vi "Clear Plugin.vi"(8 "error in (no error)":errorcluster, 10 "Plugin":string, 11 "Execution UI in":refnum<class "Execution UI.lvclass">) -> (0 "error out":errorcluster, 3 "Execution UI out":refnum<class "Execution UI.lvclass">)   [LabVIEW 2020, in "Execution UI.lvclass"]
uses:
  Execution UI.lvclass
  Execution UI.lvclass/Execution UI.ctl
  Framework/Plugin/Plugin.lvclass
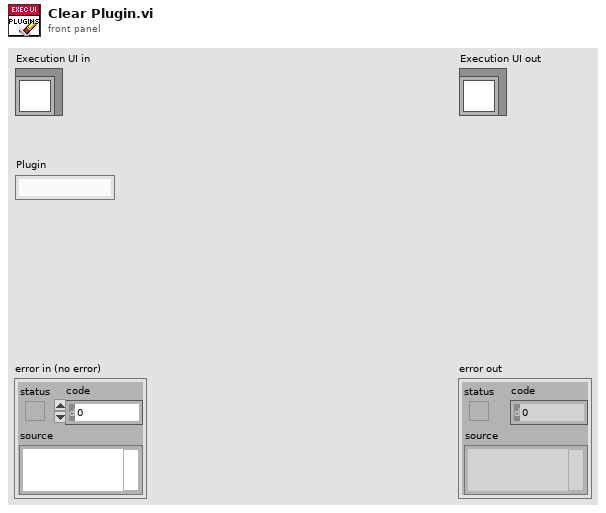
[diagram p1: front panel]
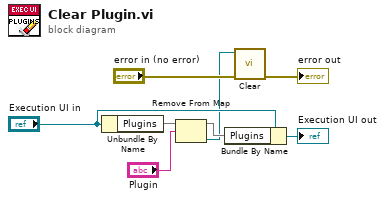
[diagram p0: block diagram]
diagram:
  n1 = Unbundle By Name("Execution UI in") -> ("Plugins"=w5:map{string, refnum<class "Plugin.lvclass">})
  n2 = Remove From Map(10:"Plugin", 11:w5) -> (1:w1:refnum<class "Plugin.lvclass">, 3:w4:map{string, refnum<class "Plugin.lvclass">})  [unwired: 1 out]
  n3 = Bundle By Name(cluster="Execution UI in", "Plugins"=w4) -> (→"Execution UI out":refnum<class "Execution UI.lvclass">)
  n4 = call-dynamic "Clear.vi"("error in (no error)"="error in (no error)", "Plugin in"=w1) -> ("error out"=→"error out":errorcluster)  [unwired: 9 in]
